vi "SetTextToBoolCtrl.vi"(10 "문자열":string, 11 "bool ref":refnum<vi>) -> ()   [LabVIEW 2018, in "Library-Ctrl.lvlib"]
uses:
  Library-Ctrl.lvlib
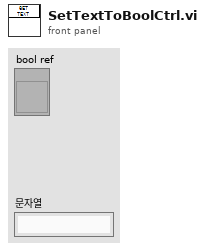
[diagram p1: front panel]
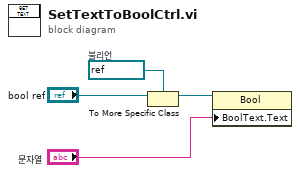
[diagram p0: block diagram]
diagram:
  w3 = refnum<vi> refnum  # 불리언
  n1 = To More Specific Class(target class=w3, reference="bool ref") -> (specific class reference=w2:refnum<vi>)  [unwired: 1 in, 1 out]
  n2 = property class="Bool"(reference=w2, "BoolText.Text"="문자열") -> ()  [unwired: 1 in, 2 out]
